vi "Get Robot Orientation.vi"(1 "Throttle In":dbl) -> (0 "Robot Orientation Out":T1)   [LabVIEW 2012]
uses:
  Controls/Robot Orientation.ctl
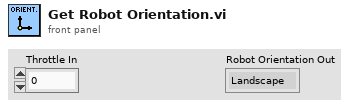
[diagram p1: front panel]
types:
  T1 = typedef "Robot Orientation.ctl" = enum16{"Landscape", "Portrait"}
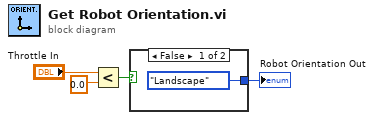
[diagram p0: block diagram]
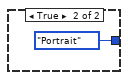
[diagram p2: hidden frame]
diagram:
  n1 = Less?(x="Throttle In", y=0.0) -> (x < y?=w2:bool)
  n2 = case shown="False" w2 {
    tunnel: [Robot_Orientation."Landscape" ("Robot Orientation") Robot_Orientation."Portrait" ("Robot Orientation")] -> w1
    frame False {
    }
    frame True {
    }
  }
  "Robot Orientation Out" <- w1
